vi "TestKeithley.vi"() -> ()   [LabVIEW 2018]
uses:
  Channel.ctl
  Keithley 2600 Series.lvlib
panel:
  out "Bottom Coil (W)":string
  out "Top Coil (W)":string
  out "Heater Error":errorcluster
  in  "stop":bool
  in  "Bottom Coil (mA)":dbl
  in  "Top Coil (mA)":dbl
  in  "Bottom Coil":bool
  in  "Top Coil":bool
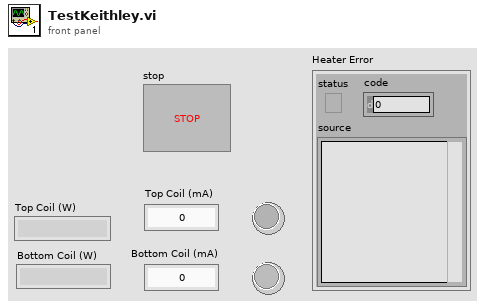
[diagram p1: front panel]
types:
  T1 = typedef "Keithley 2600 Series.lvlib/Channel.ctl" = enum32{"Channel A", "Channel B"}
  T2 = enum32{"Current", "Voltage", "IV", "Resistance", "Power"}
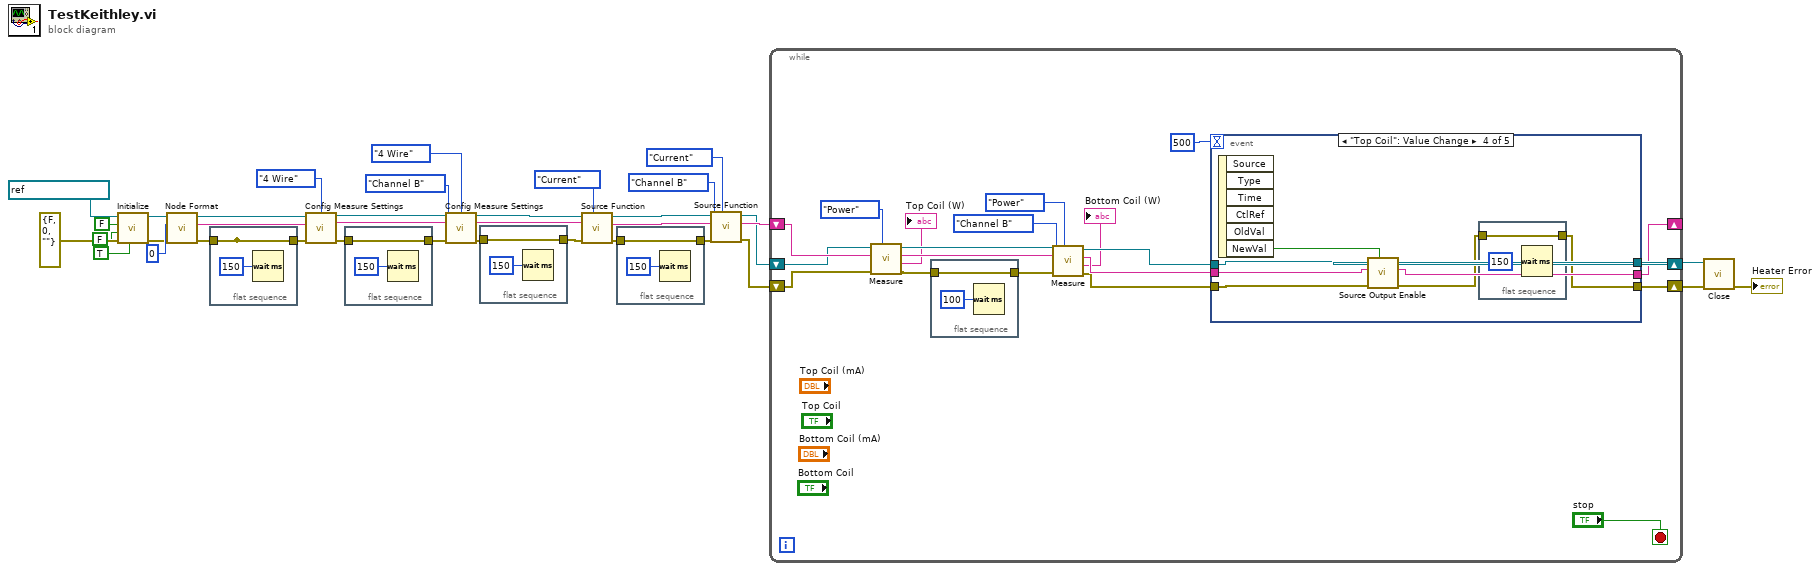
[diagram p0: block diagram]
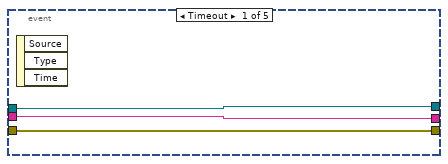
[diagram p2: hidden frame]
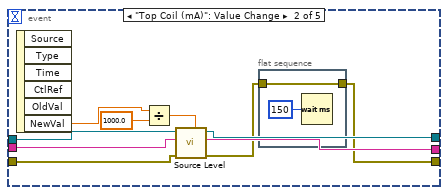
[diagram p3: hidden frame]
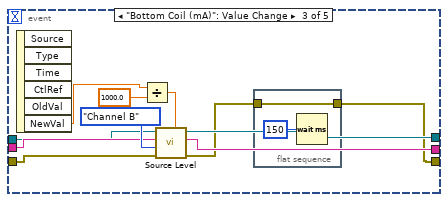
[diagram p4: hidden frame]
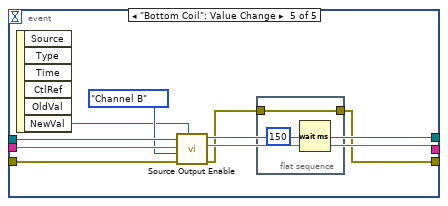
[diagram p5: hidden frame]
diagram:
  n1 = call "Initialize.vi"("Reset (True)"=TRUE, "error in (no error)"=errorcluster {"status"=FALSE, "code"=0, "source"=""}, "Error Query (False)"=FALSE, "ID Query (True)"=FALSE, "VISA resource name"=refnum<visa-resource-name> "Keithley2614B") -> ("error out"=w19:errorcluster, "VISA resource name out"=w33:refnum<visa-resource-name>)  [unwired: 5 in]
  n2 = call "Node Format.vi"("error in"=w19, "Node (0-64)"=i8 0) -> ("error out"=w8:errorcluster, "Formatted Node"=w23:string)  [unwired: 8 in]
  n3 = flat-sequence {
    tunnel: w8 -> [w36]
    tunnel: [w36] -> _
    tunnel: [w36] -> w7
    frame #0 {
      n4 = Wait (ms)(milliseconds to wait=u32 150) -> ()  [unwired: 1 out]
    }
  }
  n5 = call "Config Measure Settings.vi"("VISA resource name"=w33, "Sense (2 Wire)"=enum32{"2 Wire", "4 Wire", "Calibration"}."4 Wire", "Node In"=w23, "error in"=w7) -> ("VISA resource name out"=w30:refnum<visa-resource-name>, "Node Out"=w22:string, "error out"=w6:errorcluster)  [unwired: 8 in, 1 out]
  n6 = flat-sequence {
    tunnel: w6 -> [w38]
    tunnel: [w38] -> w5
    frame #0 {
      n7 = Wait (ms)(milliseconds to wait=u32 150) -> ()  [unwired: 1 out]
    }
  }
  n8 = call "Config Measure Settings.vi"("VISA resource name"=w30, "Sense (2 Wire)"=enum32{"2 Wire", "4 Wire", "Calibration"}."4 Wire", "Node In"=w22, "Channel (Channel A)"=Channel."Channel B", "error in"=w5) -> ("VISA resource name out"=w29:refnum<visa-resource-name>, "Node Out"=w21:string, "error out"=w4:errorcluster)  [unwired: 7 in, 1 out]
  n9 = flat-sequence {
    tunnel: w4 -> [w40]
    tunnel: [w40] -> w3
    frame #0 {
      n10 = Wait (ms)(milliseconds to wait=u32 150) -> ()  [unwired: 1 out]
    }
  }
  n11 = call "Source Function.vi"("Function (Current)"=enum32{"Current", "Voltage"}."Current", "error in (no error)"=w3, "Node In"=w21, "VISA resource name"=w29) -> ("error out"=w2:errorcluster, "Node Out"=w20:string, "VISA resource name out"=w28:refnum<visa-resource-name>)  [unwired: 4 in, 1 out]
  n12 = flat-sequence {
    tunnel: w2 -> [w42]
    tunnel: [w42] -> w1
    frame #0 {
      n13 = Wait (ms)(milliseconds to wait=u32 150) -> ()  [unwired: 1 out]
    }
  }
  n14 = call "Source Function.vi"("Function (Current)"=enum32{"Current", "Voltage"}."Current", "error in (no error)"=w1, "Channel (Channel A)"=Channel."Channel B", "Node In"=w20, "VISA resource name"=w28) -> ("error out"=w14:errorcluster, "Node Out"=w13:string, "VISA resource name out"=w12:refnum<visa-resource-name>)  [unwired: 3 in, 1 out]
  n15 = while {
    shift-right: [w62] -> _
    shift-left: w13 -> [w58]
    shift-right: [w63] -> w10
    shift-left: w12 -> [w57]
    shift-right: [w61] -> w9
    shift-left: w14 -> [w56]
    stop <- "stop" stop-if-true
    n16 = call "Measure.vi"("Function (Current)"=T2."Power", "error in (no error)"=w56, "Node In"=w58, "VISA resource name"=w57) -> ("error out"=w49:errorcluster, "Output"=→"Top Coil (W)":string, "Node Out"=w50:string, "VISA resource name out"=w51:refnum<visa-resource-name>)  [unwired: 3 in, 1 out]
    n17 = flat-sequence {
      tunnel: w49 -> [w64]
      tunnel: [w64] -> w48
      frame #0 {
        n18 = Wait (ms)(milliseconds to wait=u32 100) -> ()  [unwired: 1 out]
      }
    }
    n19 = call "Measure.vi"("Function (Current)"=T2."Power", "error in (no error)"=w48, "Channel (Channel A)"=Channel."Channel B", "Node In"=w50, "VISA resource name"=w51) -> ("error out"=w53:errorcluster, "Output"=→"Bottom Coil (W)":string, "Node Out"=w54:string, "VISA resource name out"=w55:refnum<visa-resource-name>)  [unwired: 2 in, 1 out]
    n20 = event shown="[3] \"Top Coil\": Value Change" {
      selector: _ -> [_ _ _ _ _]
      dyn-events: _ -> [_ _ _ _ _]
      timeout: 500 -> [_ _ _ _ _]
      tunnel: w54 -> [w67 w77 w87 w98 w109]
      tunnel: w53 -> [w66 w78 w90 w101 w112]
      tunnel: w55 -> [w68 w76 w86 w97 w108]
      tunnel: [w68 w75 w88 w99 w110] -> w63
      tunnel: [w67 w74 w89 w100 w111] -> w62
      tunnel: [w66 w69 w81 w94 w104] -> w61
      event Timeout {
        n21 = event-data() -> ()  [unwired: 1 in, 3 out]
      }
      event "Top Coil (mA)": Value Change {
        n22 = event-data() -> ("NewVal"=w72:dbl)  [unwired: 1 in, 5 out]
        n23 = Divide(x=w72, y=1000.0) -> (x/y=w71:dbl)
        n24 = call "Source Level.vi"("Level (0.000)"=w71, "error in (no error)"=w78, "Node In"=w77, "VISA resource name"=w76) -> ("error out"=w70:errorcluster, "Node Out"=w74:string, "VISA resource name out"=w75:refnum<visa-resource-name>)  [unwired: 4 in, 1 out]
        n25 = flat-sequence {
          tunnel: w70 -> [w79]
          tunnel: [w79] -> w69
          frame #0 {
            n26 = Wait (ms)(milliseconds to wait=u32 150) -> ()  [unwired: 1 out]
          }
        }
      }
      event "Bottom Coil (mA)": Value Change {
        n27 = event-data() -> ("NewVal"=w84:dbl)  [unwired: 1 in, 5 out]
        n28 = Divide(x=w84, y=1000.0) -> (x/y=w83:dbl)
        n29 = call "Source Level.vi"("Level (0.000)"=w83, "error in (no error)"=w90, "Channel (Channel A)"=Channel."Channel B", "Node In"=w87, "VISA resource name"=w86) -> ("error out"=w82:errorcluster, "Node Out"=w89:string, "VISA resource name out"=w88:refnum<visa-resource-name>)  [unwired: 3 in, 1 out]
        n30 = flat-sequence {
          tunnel: w82 -> [w92]
          tunnel: [w92] -> w81
          frame #0 {
            n31 = Wait (ms)(milliseconds to wait=u32 150) -> ()  [unwired: 1 out]
          }
        }
      }
      event "Top Coil": Value Change {
        n32 = event-data() -> ("NewVal"=w96:bool)  [unwired: 1 in, 5 out]
        n33 = call "Source Output Enable.vi"("Output (Off)"=w96, "error in (no error)"=w101, "Node In"=w98, "VISA resource name"=w97) -> ("error out"=w95:errorcluster, "Node Out"=w100:string, "VISA resource name out"=w99:refnum<visa-resource-name>)  [unwired: 4 in, 1 out]
        n34 = flat-sequence {
          tunnel: w95 -> [w102]
          tunnel: [w102] -> w94
          frame #0 {
            n35 = Wait (ms)(milliseconds to wait=u32 150) -> ()  [unwired: 1 out]
          }
        }
      }
      event "Bottom Coil": Value Change {
        n36 = event-data() -> ("NewVal"=w106:bool)  [unwired: 1 in, 5 out]
        n37 = call "Source Output Enable.vi"("Output (Off)"=w106, "error in (no error)"=w112, "Channel (Channel A)"=Channel."Channel B", "Node In"=w109, "VISA resource name"=w108) -> ("error out"=w105:errorcluster, "Node Out"=w111:string, "VISA resource name out"=w110:refnum<visa-resource-name>)  [unwired: 3 in, 1 out]
        n38 = flat-sequence {
          tunnel: w105 -> [w113]
          tunnel: [w113] -> w104
          frame #0 {
            n39 = Wait (ms)(milliseconds to wait=u32 150) -> ()  [unwired: 1 out]
          }
        }
      }
    }
  }
  n40 = call "Close.vi"("error in (no error)"=w9, "VISA resource name"=w10) -> ("error out"=→"Heater Error":errorcluster)  [unwired: 9 in]
